vi "S2C_M2p5942_Proc_Initialize.vi"(7 "Local?":bool, 8 "Error In":errorcluster, 10 "Command":string, 11 "JSON String":string) -> (0 "Error Out":errorcluster, 3 "Response":string)   [LabVIEW 2024]
uses:
  S2C_M2p5942_Proc_Globals.vi
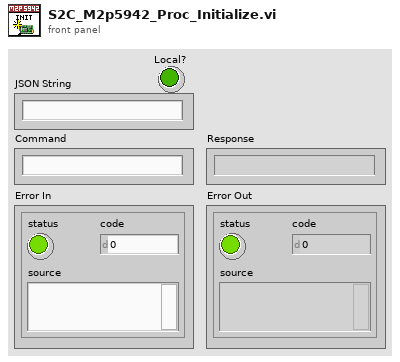
[diagram p1: front panel]
types:
  T1 = cluster{"Index":u32, "IP Address":string, "Device":u16}
  T2 = cluster{"Card Type":i32, "Inst Mem (high part)":i32, "Inst Mem (low part)":i32, "Serial Number":i32, "Function Type":i32, "Installed Features":i32, "Base Card Version":i32, "Module Version":i32, "Extension Version":i32, "Production Date":i32, "Max Sampling Rate":i32, "Max Channels":i32, "Demo Card":i32}
  T3 = cluster{"AI Channels":i32, "AI Ranges":i32, "Input Ranges (mV)":i32[], "Programmable Offset":i32, "Termination Available":bool, "SE/Diff switchable":bool, "Offset in per cent/mV":bool, "Offset Calibration":bool, "Gain Calibration":bool, "Offset with open inputs":bool, "AI Range Strings[]":string[], "Bit Resolution":i32, "AC Coupling available":bool, "BW Limit available":bool, "AI Path count":i32}
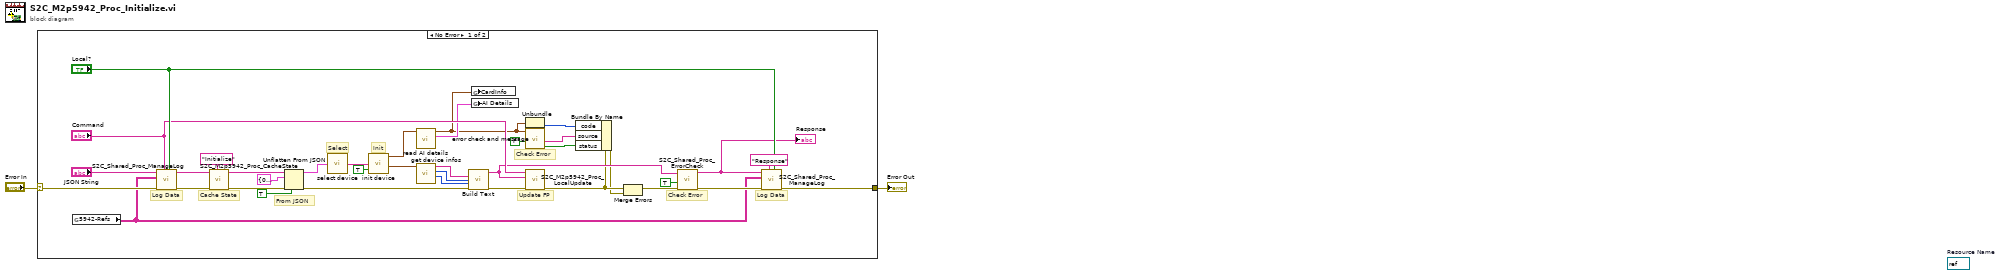
[diagram p0: block diagram]
diagram:
  (unwired) refnum<visa-resource-name> refnum  # Resource Name
  n1 = case shown="No Error" "Error In" {
    selector: "Error In" -> [w38 w40]
    tunnel: [w36 w40] -> w1
    frame No Error {
      # "Check Error"
      # "Update FP"
      # "Init"
      # "Select"
      # "Check Error"
      # "Cache State"
      # "Log Data"
      # "Log Data"
      # "From JSON"
      n2 = global read "S2C_M2p5942_Proc_Globals.vi" "5942-Refs"() -> (w20:string[][])
      n3 = call "S2C_Shared_Proc_ManageLog.vi"("Local?"="Local?", "Command"="Command", "Error In"=w38, "Refs"=w20, "Data In"="JSON String") -> ("Error Out"=w34:errorcluster, "Data Out"=w33:string)  [unwired: 5 in]
      n4 = call "S2C_M2p5942_Proc_CacheState.vi"("Label"="Initialize", "Error In"=w34, "Data In"=w33) -> ("Error Out"=w31:errorcluster, "Data Out"=w32:string)  [unwired: 7 in]
      n5 = Unflatten From JSON(JSON string=w32, type and defaults=T1 {"Index"=0, "IP Address"="", "Device"=0} ("Initialize"), default null elements? (F)=TRUE, error in (no error)=w31) -> (value=w25:T1, error out=w19:errorcluster)  [unwired: 3 in]
      n6 = call "select device.vi"("Device"=w25) -> ("device string"=w24:string)  [unwired: 4 in]
      n7 = call "init device.vi"("Device String"=w24, "Free All Devices"=TRUE) -> ("Card Info Out"=w22:cluster{"Card Handle":u64, "Error Code":u32}, "Card Information"=w21:T2)  [unwired: 3 in]
      n8 = call "read AI details.vi"("Card Info In"=w22) -> ("AI Details"=w13:T3, "Card Info Out"=w4:cluster{"Card Handle":u64, "Error Code":u32})  [unwired: 5 in]
      n9 = call "get device infos.vi"("Card Information"=w21) -> ("Mem (MB)"=w18:i32, "SN"=w17:i32, "Card Name"=w16:string)  [unwired: 8 in]
      n10 = call "Build Text"("Name"=w16, "SN"=w17, "Mem"=w18, "error in (no error)"=w19) -> ("Result"=w10:string, "error out"=w15:errorcluster)  [unwired: 10 in]
      n11 = global write "S2C_M2p5942_Proc_Globals.vi" "CardInfo"(w4) -> ()
      n12 = global write "S2C_M2p5942_Proc_Globals.vi" "AI Details"(w13) -> ()
      n13 = Unbundle(w4) -> ("Error Code"=w3:u32)  [unwired: 1 out]
      n14 = call "error check and message.vi"("Display Message (true)"=FALSE, "Card Info In"=w4) -> ("Error occurred"=w12:bool, "Error Message"=w11:string)  [unwired: 3 in, 1 out]
      n15 = call "S2C_M2p5942_Proc_LocalUpdate.vi"("Error In"=w15, "Data"=w10, "Command"="Command") -> ("Error Out"=w7:errorcluster)  [unwired: 8 in]
      n16 = Bundle By Name(cluster=w7, "code"=w3, "source"=w11, "status"=w12) -> (w6:errorcluster)
      n17 = Merge Errors(w7, w6) -> (w5:errorcluster)
      n18 = call "S2C_Shared_Proc_ErrorCheck.vi"("Error In"=w5, "ExpReply?"=TRUE, "Reply Text"=w10) -> ("Error Out"=w28:errorcluster, "Status"=w9:string)  [unwired: 7 in]
      "Response" <- w9
      n19 = call "S2C_Shared_Proc_ManageLog.vi"("Local?"="Local?", "Command"="Response", "Error In"=w28, "Refs"=w20, "Data In"=w9) -> ("Error Out"=w36:errorcluster)  [unwired: 5 in, 1 out]
    }
    frame Error {
    }
  }
  "Error Out" <- w1
